vi "acc count.vi"(6 "i":i32, 8 "time":dbl, 9 "斜":dbl, 10 "高":dbl, 11 "面積":dbl) -> (0 "stop":bool, 1 "保持時間":dbl, 2 "s":dbl, 3 "加減速時間":dbl)   [LabVIEW 2019]
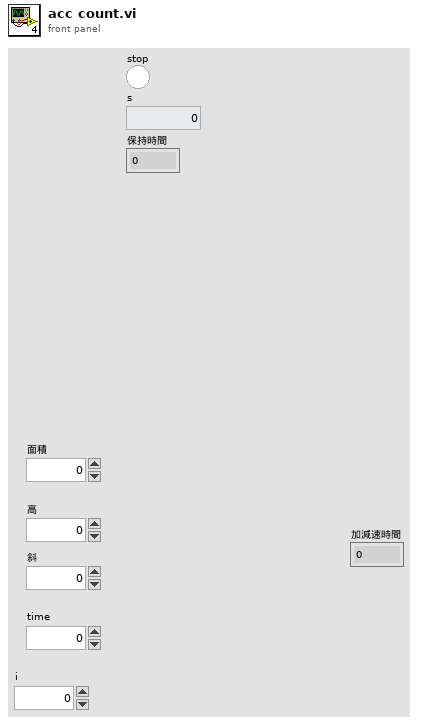
[diagram p1: front panel]
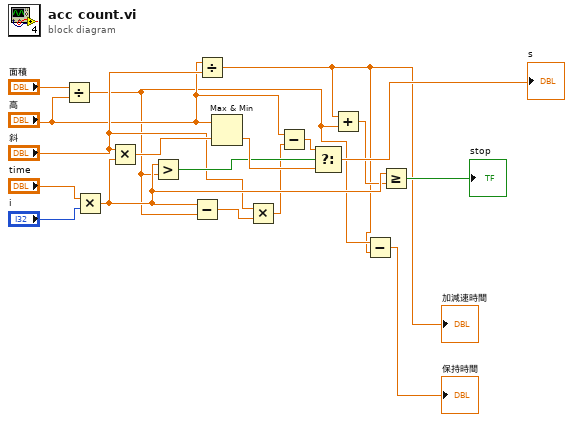
[diagram p0: block diagram]
diagram:
  n1 = Divide(x="面積", y="高") -> (x/y=w3:dbl)
  n2 = Multiply(x="time", y="i") -> (x*y=w12:dbl)
  n3 = Multiply(x="斜", y=w12) -> (x*y=w15:dbl)
  n4 = Greater?(x=w12, y=w3) -> (0:w13:bool)
  n5 = Subtract(x=w12, y=w3) -> (x-y=w10:dbl)
  n6 = Divide(x="高", y="斜") -> (x/y=w2:dbl)
  "加減速時間" <- w2
  n7 = Max & Min(x="高", y=w15) -> (min(x,y)=w14:dbl)  [unwired: 1 out]
  n8 = Multiply(x="斜", y=w10) -> (x*y=w6:dbl)
  n9 = Subtract(x="高", y=w6) -> (x-y=w8:dbl)
  n10 = Select(t=w8, s=w13, f=w14) -> (s? t:f=→"s":dbl)
  n11 = Add(x=w2, y=w3) -> (x+y=w4:dbl)
  n12 = Subtract(x=w3, y=w2) -> (x-y=→"保持時間":dbl)
  n13 = Greater Or Equal?(x=w12, y=w4) -> (x >= y?=→"stop":bool)
